vi "Get UDV Page from System Definition.vi"(8 "error in (no error)":errorcluster, 11 "System Definition Path":path) -> (0 "error out":errorcluster, 3 "NodeID":u64)   [LabVIEW 2017, in "Scan Engine EtherCAT System Tests.lvclass"]
uses:
  Scan Engine EtherCAT System Tests.lvclass
  NationalInstruments.VeriStand.SystemDefinitionAPI
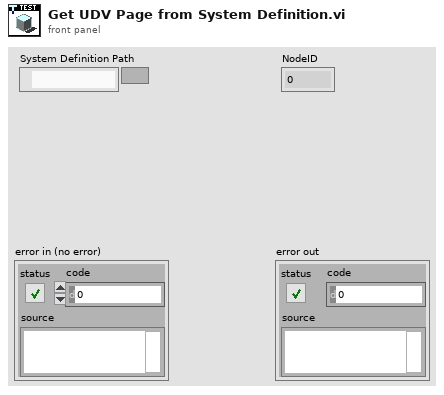
[diagram p1: front panel]
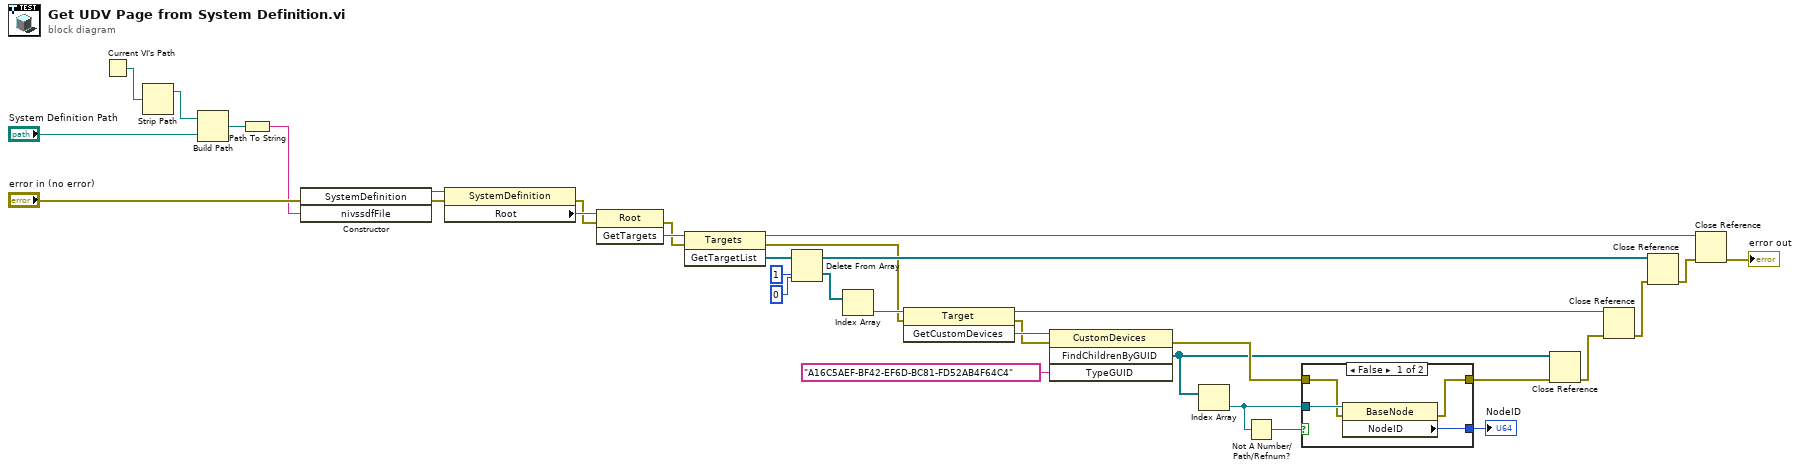
[diagram p0: block diagram]
diagram:
  n1 = Current VI's Path() -> (path=w11:path)
  n2 = Strip Path(path=w11) -> (stripped path=w10:path)  [unwired: 1 out]
  n3 = Build Path(base path=w10, name or relative path="System Definition Path") -> (appended path=w18:path)
  n4 = Path To String(path=w18) -> (string=w20:string)
  n5 = constructor class="SystemDefinition"(error in="error in (no error)", "nivssdfFile"=w20) -> (reference out=w23:refnum<k24>, error out=w22:errorcluster)  [unwired: 2 in, 2 out]
  n6 = property class="SystemDefinition"(reference=w23, error in=w22) -> (error out=w24:errorcluster, "Root"=w25:refnum<k24>)  [unwired: 1 out]
  n7 = invoke class="Root" method="GetTargets"(reference=w25, error in=w24) -> (error out=w26:errorcluster, "GetTargets"=w27:refnum<k24>)  [unwired: 1 in, 1 out]
  n8 = invoke class="Targets" method="GetTargetList"(reference=w27, error in=w26) -> (reference out=w33:refnum<k24>, error out=w9:errorcluster, "GetTargetList"=w28:refnum<k24>[])  [unwired: 1 in]
  n9 = Delete From Array(array=w28, length=1, index=0) -> (deleted portion=w34:refnum<k24>[], array with subset deleted=w31:refnum<k24>[])
  n10 = Index Array(array=w34) -> (element=w17:refnum<k24>)  [unwired: 1 in]
  n11 = invoke class="Target" method="GetCustomDevices"(reference=w17, error in=w9) -> (reference out=w7:refnum<k24>, error out=w8:errorcluster, "GetCustomDevices"=w16:refnum<k24>)  [unwired: 1 in]
  n12 = invoke class="CustomDevices" method="FindChildrenByGUID"(reference=w16, error in=w8, "TypeGUID"="A16C5AEF-BF42-EF6D-BC81-FD52AB4F64C4") -> (error out=w6:errorcluster, "FindChildrenByGUID"=w5:refnum<k24>[])  [unwired: 1 in, 2 out]
  n13 = Index Array(array=w5) -> (element=w13:refnum<k24>)  [unwired: 1 in]
  n14 = Not A Number/Path/Refnum?(number/path/refnum=w13) -> (NaN/Path/Refnum?=w14:bool)
  n15 = case shown="False" w14 {
    tunnel: w13 -> [w38 _]
    tunnel: [w37 _] -> w12
    tunnel: w6 -> [w36 w39]
    tunnel: [w35 w39] -> w4
    frame False {
      n16 = property class="BaseNode"(reference=w38, error in=w36) -> (error out=w35:errorcluster, "NodeID"=w37:u64)  [unwired: 1 out]
    }
    frame True {
    }
  }
  "NodeID" <- w12
  n17 = Close Reference(reference=w5, error in (no error)=w4) -> (error out=w3:errorcluster)
  n18 = Close Reference(reference=w7, error in (no error)=w3) -> (error out=w2:errorcluster)
  n19 = Close Reference(reference=w31, error in (no error)=w2) -> (error out=w32:errorcluster)
  n20 = Close Reference(reference=w33, error in (no error)=w32) -> (error out=→"error out":errorcluster)
